vi "Open Conn and Read.vi"(8 "error in (no error)":errorcluster, 11 "String":string) -> (0 "error out":errorcluster, 1 "Returned String":string, 2 "Returned Error":bool, 3 "TCP Network Connection out":refnum<k5>)   [LabVIEW 2024]
doc: "This software is licensed for use under the “MIT License\"\nCopyright (c) 2019 Scott Hannahs, sth@alum.mit.edu\n\nPermission is hereby granted, free of charge, to any person obtaining a copy of this software and associated documentation files (the \"Software\"), to deal in the Software without restriction, including without limitation the rights to use, copy, modify, merge, publish, distribute, sublicense, and/or sell copies of the Software, and to permit persons to whom the Software is furnished to do so, subject to the following conditions: The above copyright notice and this permission notice shall be included in all copies or substantial portions of the Software.\n\nTHE SOFTWARE IS PROVIDED \"AS IS\", WITHOUT WARRANTY OF ANY KIND, EXPRESS OR IMPLIED, INCLUDING BUT NOT LIMITED TO THE WARRANTIES OF MERCHANTABILITY, FITNESS FOR A PARTICULAR PURPOSE AND NONINFRINGEMENT. IN NO EVENT SHALL THE AUTHORS OR COPYRIGHT HOLDERS BE LIABLE FOR ANY CLAIM, DAMAGES OR OTHER LIABILITY, WHETHER IN AN ACTION OF CONTRACT, TORT OR OTHERWISE, ARISING FROM, OUT OF OR IN CONNECTION WITH THE SOFTWARE OR THE USE OR OTHER DEALINGS IN THE SOFTWARE."
uses:
  SubVIs/Interlock 32T Net Client Globals.vi
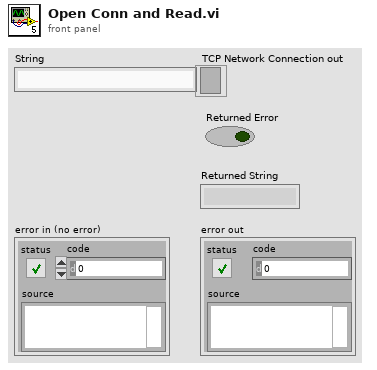
[diagram p1: front panel]
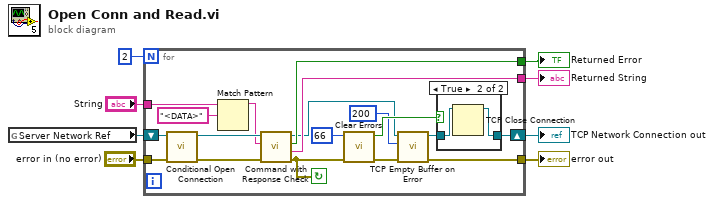
[diagram p0: block diagram]
diagram:
  n1 = global read "Interlock 32T Net Client Globals.vi" "Server Network Ref"() -> (w2:refnum<k5>)
  n2 = for {
    N: 2 -> [_]
    tunnel: [w23] -> w6
    tunnel: "String" -> [w11]
    tunnel: [w22] -> w4
    shift-right: [w17] -> w1
    shift-left: w2 -> [w18]
    tunnel: "error in (no error)" -> [w26]
    tunnel: [w15] -> w5
    stop <- w21 continue-if-true
    n3 = call "Conditional Open Connection.vi"("error in (no error)"=w26, "TCP Network Connection in"=w18) -> ("error out"=w25:errorcluster, "TCP Network Connection out"=w24:refnum<k5>)  [unwired: 8 in]
    n4 = Match Pattern(string=w11, regular expression="<DATA>") -> (before substring=w9:string)  [unwired: 1 in, 3 out]
    n5 = call "Command with Response Check.vi"("error in (no error)"=w25, "Data"=w9, "TCP Network Connection in"=w24) -> ("error out"=w21:errorcluster, "Returned String"=w22:string, "Returned Error"=w23:bool, "TCP Network Connection out"=w14:refnum<k5>)  [unwired: 5 in]
    n6 = call <vilib>:"Clear Errors.vi"("error in (no error)"=w21, "specific error code to clear (0: all)"=66) -> ("error out"=w16:errorcluster, "specific error cleared?"=w19:bool)  [unwired: 4 in]
    n7 = call "TCP Empty Buffer on Error.vi"("Error In"=w16, "timeout ms (1000)"=200, "TCP Network Connection in"=w14) -> ("Error Out"=w15:errorcluster, "TCP Network Connection out"=w13:refnum<k5>)  [unwired: 6 in, 1 out]
    n8 = case shown="True" w19 {
      tunnel: [w27 w29] -> w17
      tunnel: w13 -> [w27 w28]
      frame False {
      }
      frame True {
        n9 = TCP Close Connection(connection ID=w28) -> (connection ID out=w29:refnum<k5>)  [unwired: 2 in, 1 out]
      }
    }
  }
  "Returned Error" <- w6
  "error out" <- w5
  "TCP Network Connection out" <- w1
  "Returned String" <- w4
